vi "KonfigSeriell.vi"(1 "KonfigSeriell":T6) -> (0 "KonfigSeriell":errorcluster)   [LabVIEW 2010]
uses:
  <vilib>/LabVIEW Targets/FPGA/cRIO/shared/nicrio_ModuleControls/nicrio_cRIO-9871_XcvrModeEnum.ctl
  <vilib>/eio/EIOPropertyNode/EIOPropertyNode.xnode
  <vilib>/eio/EIOMethodNode/EIOMethodNode.xnode
  <vilib>/LabVIEW Targets/FPGA/cRIO/shared/nicrio_ModuleControls/nicrio_cRIO-9871_BaudRateEnum.ctl
  <vilib>/LabVIEW Targets/FPGA/cRIO/shared/nicrio_ModuleControls/nicrio_cRIO-9871_DataBitsEnum.ctl
  <vilib>/LabVIEW Targets/FPGA/cRIO/shared/nicrio_ModuleControls/nicrio_cRIO-9871_ParityEnum.ctl
  <vilib>/LabVIEW Targets/FPGA/cRIO/shared/nicrio_ModuleControls/nicrio_cRIO-9871_StopBitsEnum.ctl
  <vilib>/LabVIEW Targets/FPGA/cRIO/shared/nicrio_ModuleControls/nicrio_cRIO-9871_FlowControlEnum.ctl
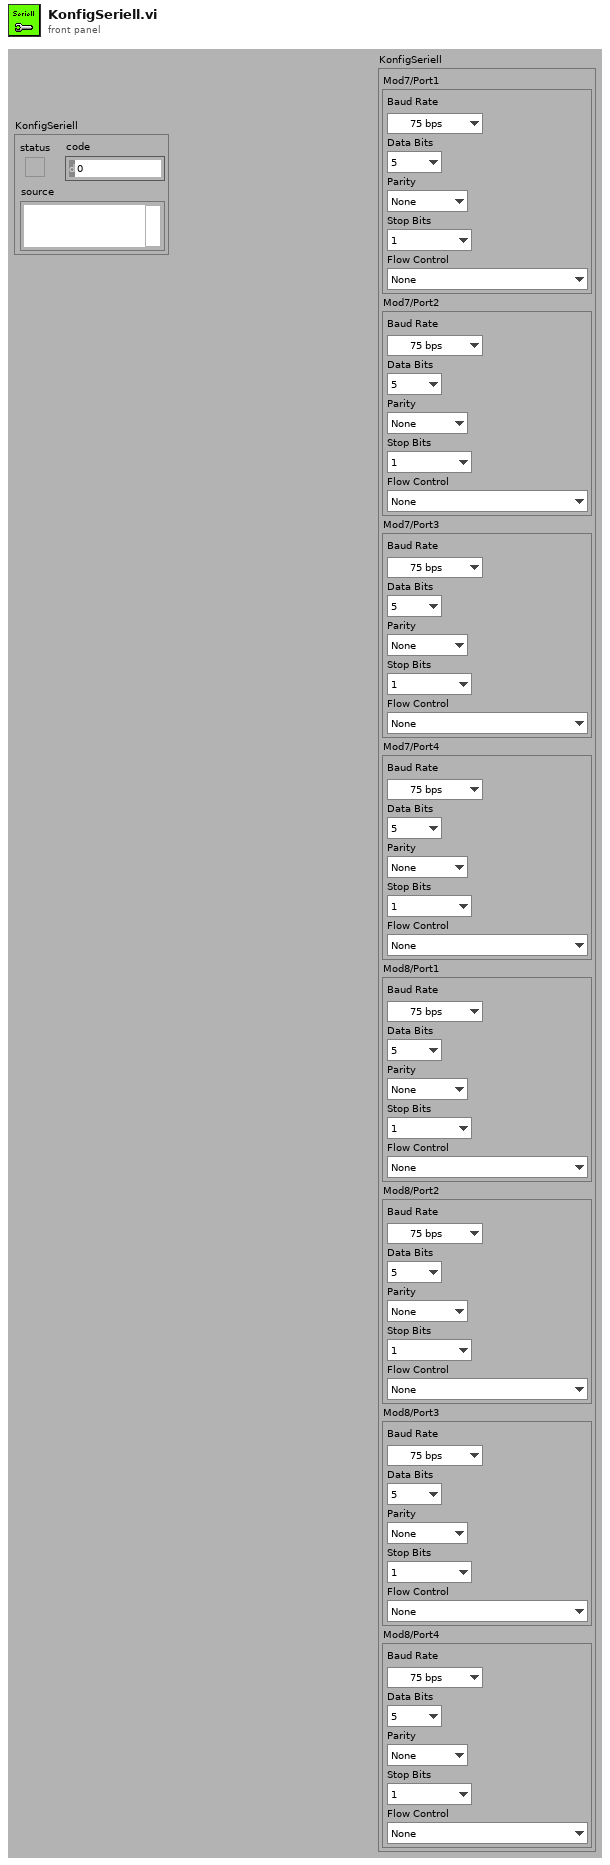
[diagram p1: front panel]
types:
  T1 = typedef "nicrio_cRIO-9871_BaudRateEnum.ctl" = enum16{"75 bps", "110 bps", "134 bps", "150 bps", "300 bps", "600 bps", "1200 bps", "1800 bps", "2400 bps", "4800 bps", "7200 bps", "9600 bps", "14.4 kbps", "19.2 kbps", "28.8 kbps", "38.4 kbps", "57.6 kbps", "115.2 kbps", "230.4 kbps", "460.8 kbps", "921.6 kbps"}
  T2 = typedef "nicrio_cRIO-9871_DataBitsEnum.ctl" = enum8{"5", "6", "7", "8"}
  T3 = typedef "nicrio_cRIO-9871_ParityEnum.ctl" = enum8{"None", "Odd", "Even", "Mark", "Space"}
  T4 = typedef "nicrio_cRIO-9871_StopBitsEnum.ctl" = enum8{"1", "1.5", "2"}
  T5 = typedef "nicrio_cRIO-9871_FlowControlEnum.ctl" = enum8{"None", "Software (XON / XOFF)", "Hardware (RTS / CTS)"}
  T6 = cluster{"Mod7/Port1":cluster{"Baud Rate":T1, "Data Bits":T2, "Parity":T3, "Stop Bits":T4, "Flow Control":T5}, "Mod7/Port2":cluster{"Baud Rate":T1, "Data Bits":T2, "Parity":T3, "Stop Bits":T4, "Flow Control":T5}, "Mod7/Port3":cluster{"Baud Rate":T1, "Data Bits":T2, "Parity":T3, "Stop Bits":T4, "Flow Control":T5}, "Mod7/Port4":cluster{"Baud Rate":T1, "Data Bits":T2, "Parity":T3, "Stop Bits":T4, "Flow Control":T5}, "Mod8/Port1":cluster{"Baud Rate":T1, "Data Bits":T2, "Parity":T3, "Stop Bits":T4, "Flow Control":T5}, "Mod8/Port2":cluster{"Baud Rate":T1, "Data Bits":T2, "Parity":T3, "Stop Bits":T4, "Flow Control":T5}, "Mod8/Port3":cluster{"Baud Rate":T1, "Data Bits":T2, "Parity":T3, "Stop Bits":T4, "Flow Control":T5}, "Mod8/Port4":cluster{"Baud Rate":T1, "Data Bits":T2, "Parity":T3, "Stop Bits":T4, "Flow Control":T5}}
  T7 = typedef "nicrio_cRIO-9871_XcvrModeEnum.ctl" = enum8{"4 Wire", "2 Wire DTR Controlled with Echo", "2 Wire DTR Controlled", "2 Wire Auto"}
  T8 = cluster{"Baud Rate":T1, "Data Bits":T2, "Parity":T3, "Stop Bits":T4, "Flow Control":T5}
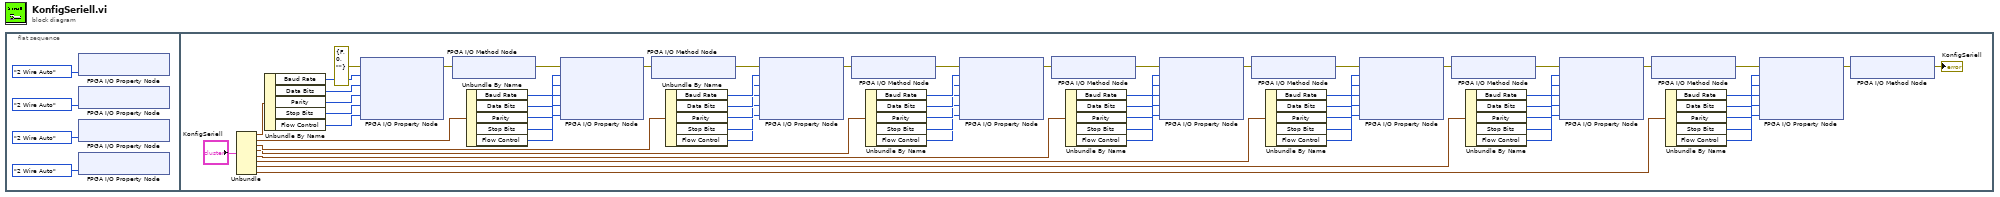
[diagram p0: block diagram]
diagram:
  n1 = flat-sequence {
    frame #0 {
      n2 = xnode "FPGA I/O Property Node"("Transceiver Mode"=nicrio_cRIO-9871_XcvrModeEnum."2 Wire Auto") -> ()  [unwired: 1 in, 1 out]
      n3 = xnode "FPGA I/O Property Node"("Transceiver Mode"=nicrio_cRIO-9871_XcvrModeEnum."2 Wire Auto") -> ()  [unwired: 1 in, 1 out]
      n4 = xnode "FPGA I/O Property Node"("Transceiver Mode"=nicrio_cRIO-9871_XcvrModeEnum."2 Wire Auto") -> ()  [unwired: 1 in, 1 out]
      n5 = xnode "FPGA I/O Property Node"("Transceiver Mode"=nicrio_cRIO-9871_XcvrModeEnum."2 Wire Auto") -> ()  [unwired: 1 in, 1 out]
    }
    frame #1 {
      n6 = Unbundle("KonfigSeriell") -> ("Mod7/Port1"=w12:T8, "Mod7/Port2"=w11:T8, "Mod7/Port3"=w10:T8, "Mod7/Port4"=w9:T8, "Mod8/Port1"=w8:T8, "Mod8/Port2"=w7:T8, "Mod8/Port3"=w6:T8, "Mod8/Port4"=w5:T8)
      n7 = Unbundle By Name(w12) -> ("Baud Rate"=w16:T1, "Data Bits"=w17:T2, "Parity"=w18:T3, "Stop Bits"=w19:T4, "Flow Control"=w20:T5)
      n8 = xnode "FPGA I/O Property Node"("error in"=errorcluster {"status"=FALSE, "code"=0, "source"=""}, "Baud Rate"=w16, "Data Bits"=w17, "Parity"=w18, "Stop Bits"=w19, "Flow Control"=w20) -> ("error out"=w36:errorcluster)  [unwired: 1 in, 1 out]
      n9 = xnode "FPGA I/O Method Node"("error in"=w36) -> ("error out"=w37:errorcluster)  [unwired: 1 in, 1 out]
      n10 = Unbundle By Name(w11) -> ("Baud Rate"=w21:T1, "Data Bits"=w22:T2, "Parity"=w23:T3, "Stop Bits"=w24:T4, "Flow Control"=w25:T5)
      n11 = xnode "FPGA I/O Property Node"("error in"=w37, "Baud Rate"=w21, "Data Bits"=w22, "Parity"=w23, "Stop Bits"=w24, "Flow Control"=w25) -> ("error out"=w38:errorcluster)  [unwired: 1 in, 1 out]
      n12 = xnode "FPGA I/O Method Node"("error in"=w38) -> ("error out"=w39:errorcluster)  [unwired: 1 in, 1 out]
      n13 = Unbundle By Name(w10) -> ("Baud Rate"=w30:T1, "Data Bits"=w29:T2, "Parity"=w28:T3, "Stop Bits"=w27:T4, "Flow Control"=w26:T5)
      n14 = xnode "FPGA I/O Property Node"("error in"=w39, "Baud Rate"=w30, "Data Bits"=w29, "Parity"=w28, "Stop Bits"=w27, "Flow Control"=w26) -> ("error out"=w40:errorcluster)  [unwired: 1 in, 1 out]
      n15 = xnode "FPGA I/O Method Node"("error in"=w40) -> ("error out"=w41:errorcluster)  [unwired: 1 in, 1 out]
      n16 = Unbundle By Name(w9) -> ("Baud Rate"=w35:T1, "Data Bits"=w34:T2, "Parity"=w33:T3, "Stop Bits"=w32:T4, "Flow Control"=w31:T5)
      n17 = xnode "FPGA I/O Property Node"("error in"=w41, "Baud Rate"=w35, "Data Bits"=w34, "Parity"=w33, "Stop Bits"=w32, "Flow Control"=w31) -> ("error out"=w42:errorcluster)  [unwired: 1 in, 1 out]
      n18 = xnode "FPGA I/O Method Node"("error in"=w42) -> ("error out"=w70:errorcluster)  [unwired: 1 in, 1 out]
      n19 = Unbundle By Name(w8) -> ("Baud Rate"=w43:T1, "Data Bits"=w44:T2, "Parity"=w45:T3, "Stop Bits"=w46:T4, "Flow Control"=w47:T5)
      n20 = xnode "FPGA I/O Property Node"("error in"=w70, "Baud Rate"=w43, "Data Bits"=w44, "Parity"=w45, "Stop Bits"=w46, "Flow Control"=w47) -> ("error out"=w48:errorcluster)  [unwired: 1 in, 1 out]
      n21 = xnode "FPGA I/O Method Node"("error in"=w48) -> ("error out"=w67:errorcluster)  [unwired: 1 in, 1 out]
      n22 = Unbundle By Name(w7) -> ("Baud Rate"=w49:T1, "Data Bits"=w50:T2, "Parity"=w51:T3, "Stop Bits"=w52:T4, "Flow Control"=w53:T5)
      n23 = xnode "FPGA I/O Property Node"("error in"=w67, "Baud Rate"=w49, "Data Bits"=w50, "Parity"=w51, "Stop Bits"=w52, "Flow Control"=w53) -> ("error out"=w54:errorcluster)  [unwired: 1 in, 1 out]
      n24 = xnode "FPGA I/O Method Node"("error in"=w54) -> ("error out"=w68:errorcluster)  [unwired: 1 in, 1 out]
      n25 = Unbundle By Name(w6) -> ("Baud Rate"=w55:T1, "Data Bits"=w56:T2, "Parity"=w57:T3, "Stop Bits"=w58:T4, "Flow Control"=w59:T5)
      n26 = xnode "FPGA I/O Property Node"("error in"=w68, "Baud Rate"=w55, "Data Bits"=w56, "Parity"=w57, "Stop Bits"=w58, "Flow Control"=w59) -> ("error out"=w60:errorcluster)  [unwired: 1 in, 1 out]
      n27 = xnode "FPGA I/O Method Node"("error in"=w60) -> ("error out"=w69:errorcluster)  [unwired: 1 in, 1 out]
      n28 = Unbundle By Name(w5) -> ("Baud Rate"=w61:T1, "Data Bits"=w62:T2, "Parity"=w63:T3, "Stop Bits"=w64:T4, "Flow Control"=w65:T5)
      n29 = xnode "FPGA I/O Property Node"("error in"=w69, "Baud Rate"=w61, "Data Bits"=w62, "Parity"=w63, "Stop Bits"=w64, "Flow Control"=w65) -> ("error out"=w66:errorcluster)  [unwired: 1 in, 1 out]
      n30 = xnode "FPGA I/O Method Node"("error in"=w66) -> ("error out"=→"KonfigSeriell":errorcluster)  [unwired: 1 in, 1 out]
    }
  }
